vi "AnalogReadContinuous.vi"() -> ()   [LabVIEW 2019]
panel:
  in  "esdaqPortInp":refnum<visa-resource-name>
  out "esdaqErrorOut":errorcluster
  out "Waveform Chart":i32(graph)
  in  "Timeout":u32
  out "Value":dbl
  in  "Channel":u32=8
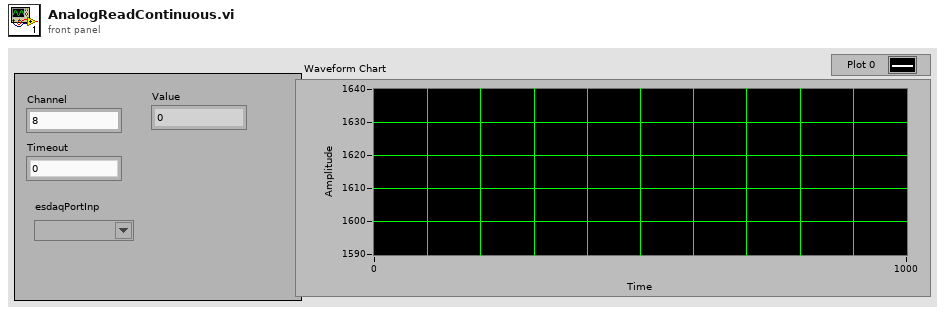
[diagram p1: front panel]
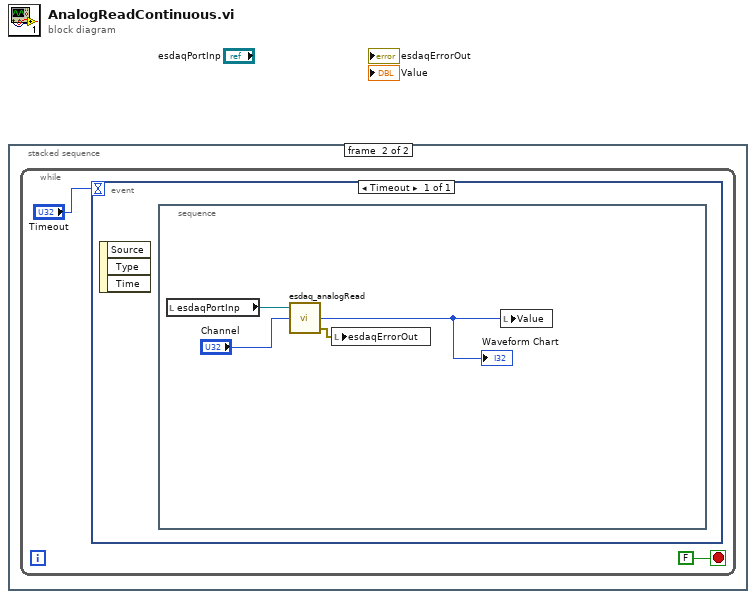
[diagram p0: block diagram]
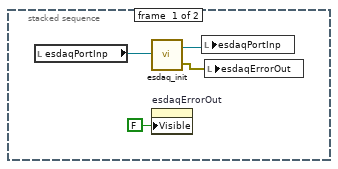
[diagram p2: hidden frame]
diagram:
  n1 = stacked-sequence {
    frame #0 {
      n2 = local read "esdaqPortInp"() -> (w3:refnum<visa-resource-name>)
      n3 = call "esdaq_init.vi"("esdaqPortInp"=w3) -> ("esdaqPortOut"=w4:refnum<visa-resource-name>, "esdaqErrorOut"=w2:errorcluster)
      n4 = property on="esdaqErrorOut" class="Clust (strict)"("Visible"=FALSE) -> ()  [unwired: 2 in, 2 out]
      n5 = local write "esdaqPortInp"(w4) -> ()
      n6 = local write "esdaqErrorOut"(w2) -> ()
    }
    frame #1 {
      n7 = while {
        stop <- FALSE stop-if-true
        n8 = event shown="[0] Timeout" {
          selector: _ -> [_]
          dyn-events: _ -> [_]
          timeout: "Timeout" -> [_]
          event Timeout {
            n9 = event-data() -> ()  [unwired: 1 in, 3 out]
            n10 = stacked-sequence {
              frame #0 {
                n11 = local read "esdaqPortInp"() -> (w9:refnum<visa-resource-name>)
                n12 = call "esdaq_analogRead.vi"("Channel"="Channel", "esdaqPortInp"=w9) -> ("esdaqErrorOut"=w10:errorcluster, "value"=w7:i32)  [unwired: 1 in, 1 out]
                "Waveform Chart" <- w7
                n13 = local write "esdaqErrorOut"(w10) -> ()
                n14 = local write "Value"(w7) -> ()
              }
            }
          }
        }
      }
    }
  }
